vi "Set Paths.vi"(7 "Measurement specific paths":T1=enum."Harmonics", 8 "error in (no error)":errorcluster, 11 "NI USB-6501 in":refnum<class "NI USB-6501.lvclass">) -> (0 "error out":errorcluster, 3 "NI USB-6501 out":refnum<class "NI USB-6501.lvclass">)   [LabVIEW 2020, in "NI USB-6501.lvclass"]
uses:
  NI USB-6501.lvclass
  Path Control/Measurements Specific Paths.ctl
  <vilib>/DAQmx/write.llb/DAQmx Write (Digital Bool 1Line 1Point).vi
  <vilib>/DAQmx/read.llb/DAQmx Read (Digital Bool 1Line 1Point).vi
  <vilib>/DAQmx/miscellaneous.llb/DAQmx Fill In Error Info.vi
  Path Control/PathControl.lvclass
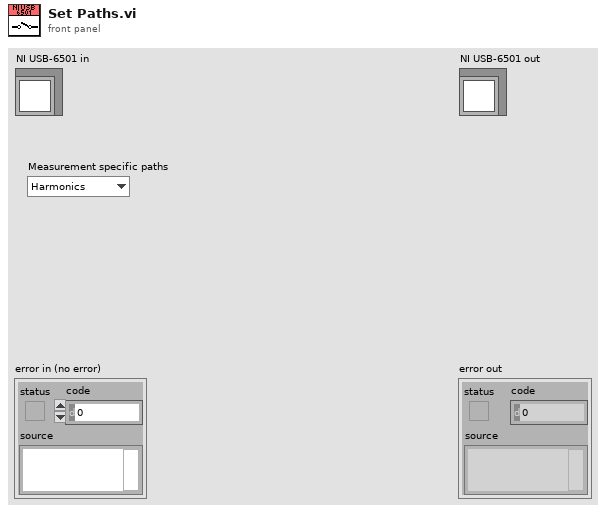
[diagram p1: front panel]
types:
  T1 = typedef "PathControl.lvclass/Measurements Specific Paths.ctl" = enum16{"No calibration", "Harmonics", "IMD", "S Parameter", "AM-AM", "MCCW-ACLR", "DC", "LCR", "Power Meter GUI", "RF Power"}
  T2 = typedef "NI USB-6501.lvclass/Channel.ctl" = cluster{"Channel":tag, "Task":refnum<k21>, "Function":string, "Low":string, "High":string, "Direction":enum16{"Input", "Output"}}
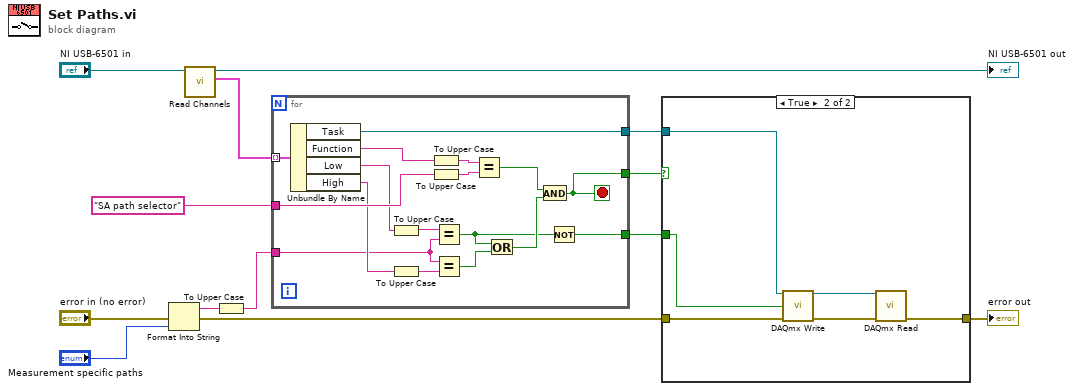
[diagram p0: block diagram]
diagram:
  n1 = Format Into String(error in="error in (no error)", "Measurement specific paths") -> (resulting string=w3:string, error out=w5:errorcluster)  [unwired: 2 in]
  n2 = call-dynamic "Read Channels.vi"("NI USB-6501 in"="NI USB-6501 in") -> ("Channels"=w11:T2[], "NI USB-6501 out"=→"NI USB-6501 out":refnum<class "NI USB-6501.lvclass">)  [unwired: 9 in]
  n3 = To Upper Case(1:w3) -> (0:w2:string)
  n4 = for {
    tunnel: w11 -> [w30] mode=indexing
    tunnel: [w29] -> w9
    tunnel: "SA path selector" ("resulting string") -> [w27]
    tunnel: [w16] -> w7
    tunnel: w2 -> [w20]
    tunnel: [w14] -> w1
    stop <- w16 stop-if-true
    n5 = Unbundle By Name(w30) -> ("Task"=w29:refnum<k21>, "Function"=w28:string, "Low"=w24:string, "High"=w23:string)
    n6 = To Upper Case(1:w24) -> (0:w21:string)
    n7 = To Upper Case(1:w23) -> (0:w22:string)
    n8 = To Upper Case(1:w28) -> (0:w26:string)
    n9 = To Upper Case(1:w27) -> (0:w25:string)
    n10 = Equal?(x=w21, y=w20) -> (x = y?=w15:bool)
    n11 = Equal?(x=w20, y=w22) -> (x = y?=w19:bool)
    n12 = Equal?(x=w26, y=w25) -> (x = y?=w17:bool)
    n13 = Or(x=w15, y=w19) -> (x .or. y?=w18:bool)
    n14 = And(x=w17, y=w18) -> (x .and. y?=w16:bool)
    n15 = Not(x=w15) -> (.not. x?=w14:bool)
  }
  n16 = case shown="True" w7 {
    tunnel: [w31 w35] -> w13
    tunnel: w5 -> [w31 w34]
    tunnel: w9 -> [_ w33]
    tunnel: w1 -> [_ w32]
    frame False {
    }
    frame True {
      n17 = call-poly <vilib>:"DAQmx Write.vi"("task/channels in"=w33, "data"=w32, "error in"=w34) -> ("task out"=w37:refnum<k21>, "error out"=w36:errorcluster)  [unwired: 10 in, 1 out]
      n18 = call-poly <vilib>:"DAQmx Read.vi"("task/channels in"=w37, "error in"=w36) -> ("error out"=w35:errorcluster)  [unwired: 11 in, 2 out]
    }
  }
  "error out" <- w13
